vi "Set All Exports.vi"(0 "Component in":refnum<class "Component.lvclass">, 5 "Exports":refnum<class "Export.lvclass">[](array[class])) -> (4 "Component out":refnum<class "Component.lvclass">)   [LabVIEW 2017, in "CL_G3_VIComponentBuilder.lvlib" / "Component.lvclass"]
doc: "Adds \\ overwrites the exports in the component."
uses:
  Component.lvclass
  Exports/Exports/Export.lvclass
  Component.lvclass/Component.ctl
  Exports/Exports/Export.lvclass/Export.ctl
  Exports/Exports/Accessors/Read unique Name.vi
  Accessors/Write Component Operations Errors.vi
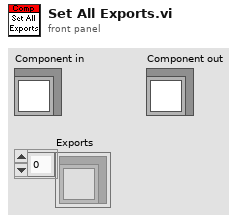
[diagram p1: front panel]
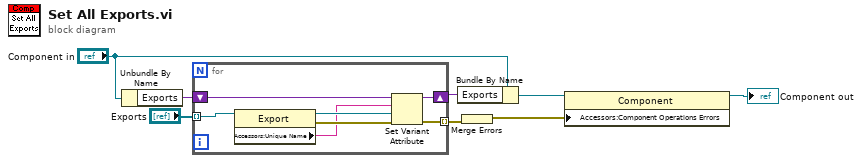
[diagram p0: block diagram]
diagram:
  n1 = Unbundle By Name("Component in") -> ("Exports"=w6:variant)
  n2 = for {
    tunnel: "Exports" -> [w13] mode=indexing
    shift-right: [w14] -> w5
    shift-left: w6 -> [w15]
    tunnel: [w11] -> w3 mode=indexing
    n3 = property class="Export"(reference=w13) -> (reference out=w12:refnum<class "Export.lvclass">, error out=w10:errorcluster, "Accessors:Unique Name"=w9:string)  [unwired: 1 in]
    n4 = Set Variant Attribute(Variant=w15, name=w9, value=w12, error in=w10) -> (Variant out=w14:variant, error out=w11:errorcluster)  [unwired: 1 out]
  }
  n5 = Bundle By Name(cluster="Component in", "Exports"=w5) -> (w4:refnum<class "Component.lvclass">)
  n6 = Merge Errors(w3) -> (w1:errorcluster)
  n7 = property class="Component"(reference=w4, "Accessors:Component Operations Errors"=w1) -> (reference out=→"Component out":refnum<class "Component.lvclass">)  [unwired: 1 in, 1 out]
